vi "SGSA_Power_Freq_Sweep_Only_ELTA.vi"() -> ()   [LabVIEW 2023, in "SG_SA.lvlib"]
uses:
  SG_SA.lvlib
  lib/Keysight/Keysight.lvlib
panel:
  out "SA Freq(MHz)":i32
  out "SG Freq(MHz)":i32
  out "[SA]_Loss":dbl=8.0
  out "[SG]_Loss":dbl=8.0
  out "SG Power":i32
  in  "[SA] -> DUT Loss\nFreq.(MHz)          Loss":dbl[][](array[numeric])
  in  "[SG] -> DUT Loss\nFreq.(MHz)       Loss":dbl[][](array[numeric])
  in  "Waiting Time(ms)":u32=100
  in  "Stop Power":i32=18
  in  "Start Power":i32=-20
  in  "AvgTimes":i32=5
  in  "FileNote":string
  in  "SG":refnum<visa-resource-name>="TCPIP0::192.168.100.201::inst0::INSTR"
  in  "SA":refnum<visa-resource-name>="TCPIP0::192.168.100.202::inst0::INSTR"
  out "Spectrum Data":cluster{"X":dbl, "Y":dbl}[](graph)
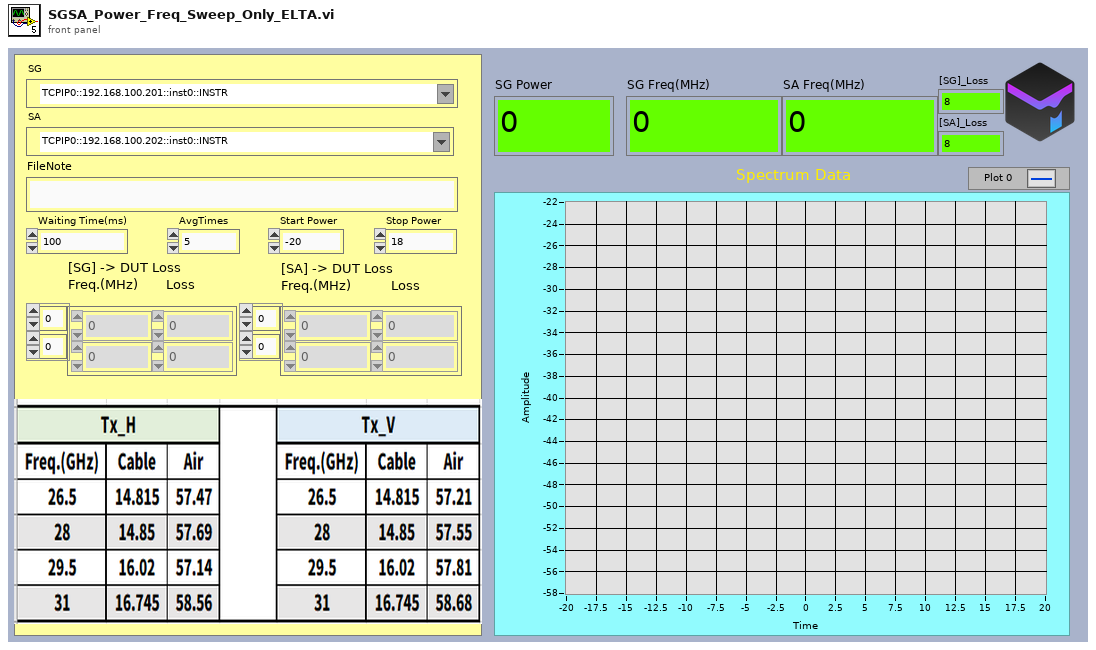
[diagram p1: front panel]
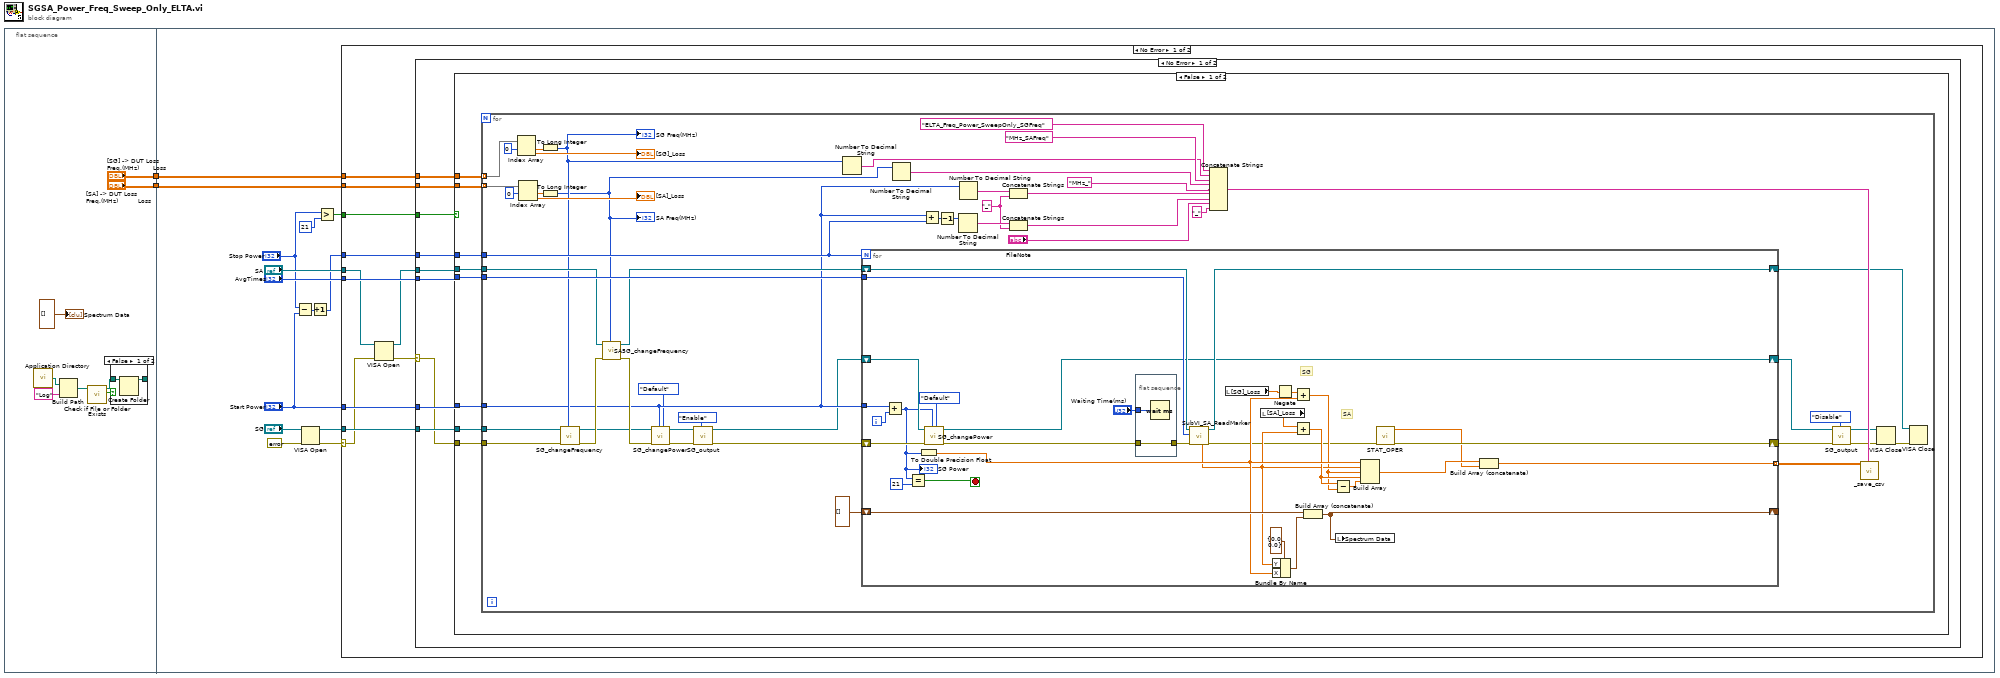
[diagram p0: block diagram]
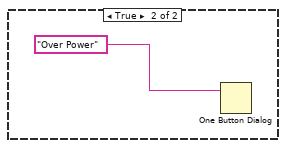
[diagram p3: hidden frame]
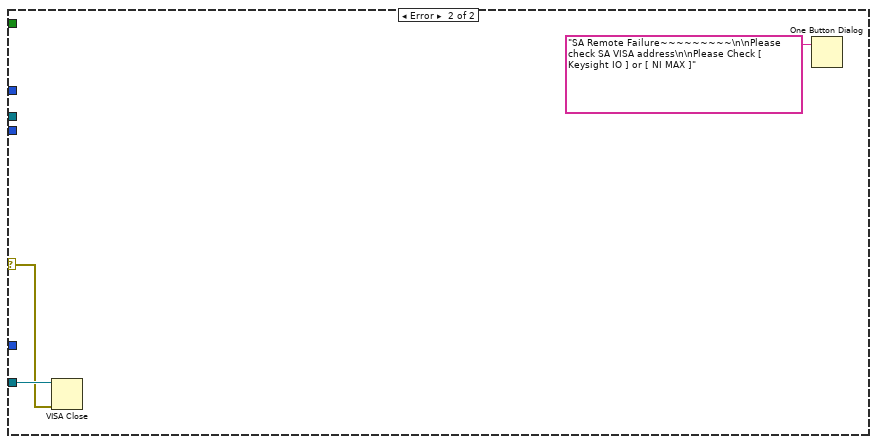
[diagram p4: hidden frame]
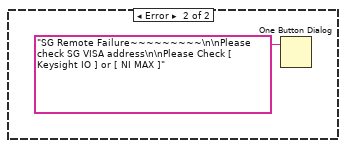
[diagram p5: hidden frame]
diagram:
  n1 = flat-sequence {
    tunnel: ["[SA] -> DUT Loss\nFreq.(MHz)          Loss"] -> w2
    tunnel: ["[SG] -> DUT Loss\nFreq.(MHz)       Loss"] -> w1
    tunnel: w2 -> [w15]
    tunnel: w1 -> [w14]
    frame #0 {
      n2 = call <vilib>:"Application Directory.vi"() -> ("Application Directory"=w9:path)
      n3 = Build Path(base path=w9, name or relative path="Log") -> (appended path=w6:path)
      n4 = call <vilib>:"Check if File or Folder Exists.vi"("path"=w6) -> ("file or folder exists?"=w8:bool, "dup path"=w7:path)  [unwired: 8 in, 1 out]
      n5 = case shown="False" w8 {
        tunnel: w7 -> [w12 w13]
        tunnel: [w11 w13] -> _
        frame False {
          n6 = Create Folder(path (use dialog)=w12) -> (created path=w11:path)  [unwired: 2 in, 2 out]
        }
        frame True {
        }
      }
      "Spectrum Data" <- cluster{"X":dbl, "Y":dbl}[] [] ("XY Graph")
    }
    frame #1 {
      n7 = Subtract(x="Stop Power", y="Start Power") -> (x-y=w23:i32)
      n8 = VISA Open(error in (no error)=errorcluster {"status"=FALSE, "code"=0, "source"=""}, VISA resource name="SG") -> (VISA resource name=w17:refnum<visa-resource-name>, error out=w16:errorcluster)  [unwired: 3 in]
      n9 = Increment(x=w23) -> (x+1=w22:i32)
      n10 = Greater?(x="Stop Power", y=21) -> (0:w26:bool)
      n11 = case shown="No Error" w16 {
        selector: w16 -> [w33 _]
        tunnel: "SA" -> [w31 _]
        tunnel: w26 -> [w38 _]
        tunnel: "Start Power" -> [w37 _]
        tunnel: "AvgTimes" -> [w36 _]
        tunnel: w22 -> [w35 _]
        tunnel: w17 -> [w34 _]
        tunnel: w15 -> [w29 _]
        tunnel: w14 -> [w28 _]
        frame No Error {
          n12 = VISA Open(error in (no error)=w33, VISA resource name=w31) -> (VISA resource name=w30:refnum<visa-resource-name>, error out=w32:errorcluster)  [unwired: 3 in]
          n13 = case shown="No Error" w32 {
            selector: w32 -> [w41 w141]
            tunnel: w30 -> [w47 _]
            tunnel: w38 -> [w46 _]
            tunnel: w37 -> [w45 _]
            tunnel: w36 -> [w44 _]
            tunnel: w35 -> [w43 _]
            tunnel: w34 -> [w42 w142]
            tunnel: w29 -> [w40 _]
            tunnel: w28 -> [w39 _]
            frame No Error {
              n14 = case shown="False" w46 {
                tunnel: w47 -> [w55 _]
                tunnel: w44 -> [w54 _]
                tunnel: w45 -> [w51 _]
                tunnel: w41 -> [w53 _]
                tunnel: w42 -> [w52 _]
                tunnel: w43 -> [w50 _]
                tunnel: w40 -> [w49 _]
                tunnel: w39 -> [w48 _]
                frame False {
                  n15 = for {
                    tunnel: w55 -> [w77]
                    tunnel: w54 -> [w105]
                    tunnel: w53 -> [w82]
                    tunnel: w52 -> [w81]
                    tunnel: w51 -> [w67]
                    tunnel: w50 -> [w96]
                    tunnel: w49 -> [w86] mode=indexing
                    tunnel: w48 -> [w89] mode=indexing
                    w100 = "_"
                    n16 = Index Array(array=w89, index #1=0 ("index")) -> (element #1=w80:dbl, element #2=→"[SG]_Loss":dbl)  [unwired: 1 in]
                    n17 = Index Array(array=w86, index #1=0 ("index")) -> (element #1=w79:dbl, element #2=→"[SA]_Loss":dbl)  [unwired: 1 in]
                    n18 = To Long Integer(number=w80) -> (32bit integer=w71:i32)
                    "SG Freq(MHz)" <- w71
                    n19 = To Long Integer(number=w79) -> (32bit integer=w70:i32)
                    "SA Freq(MHz)" <- w70
                    n20 = call "SG_changeFrequency.vi"("MHz"=w71, "error in"=w82, "VISA in"=w81) -> ("error out"=w83:errorcluster, "VISA out"=w68:refnum<visa-resource-name>)  [unwired: 6 in, 1 out]
                    n21 = call "SA5G_changeFrequency.vi"("MHz"=w70, "error in"=w83, "VISA in"=w77) -> ("error out"=w69:errorcluster, "VISA out"=w78:refnum<visa-resource-name>)  [unwired: 6 in, 1 out]
                    n22 = call "SG_changePower.vi"("Type"=enum16{"Default", "E6680A"}."Default", "dBm"=w67, "error in"=w69, "VISA in"=w68) -> ("error out"=w64:errorcluster, "VISA out"=w65:refnum<visa-resource-name>)  [unwired: 5 in, 1 out]
                    n23 = call "SG_output.vi"("Func."=enum16{"Disable", "Enable"}."Enable", "error in"=w64, "VISA in"=w65) -> ("error out"=w61:errorcluster, "VISA out"=w62:refnum<visa-resource-name>)  [unwired: 7 in]
                    n24 = Number To Decimal String(number=w71) -> (decimal integer string=w73:string)  [unwired: 1 in]
                    n25 = for {
                      N: w96 -> [_]
                      tunnel: w105 -> [w136]
                      tunnel: w67 -> [w134]
                      shift-right: [w109] -> w60
                      shift-left: w61 -> [w116]
                      shift-right: [w114] -> w59
                      shift-left: w62 -> [w113]
                      tunnel: [w107] -> w93 mode=indexing
                      shift-right: [w129] -> w90
                      shift-left: w78 -> [w137]
                      shift-right: [w125] -> _
                      shift-left: cluster{"X":dbl, "Y":dbl}[] [] ("XY Graph") -> [w127]
                      i -> [w135]
                      stop <- w132 stop-if-true
                      # "SA"
                      # "SG"
                      n26 = Add(x=w134, y=w135) -> (x+y=w112:i32)
                      "SG Power" <- w112
                      n27 = Equal?(x=w112, y=21) -> (x = y?=w132:bool)
                      n28 = To Double Precision Float(number=w112) -> (double precision float=w124:dbl)
                      n29 = call "SG_changePower.vi"("Type"=enum16{"Default", "E6680A"}."Default", "dBm"=w112, "error in"=w116, "VISA in"=w113) -> ("error out"=w115:errorcluster, "VISA out"=w114:refnum<visa-resource-name>)  [unwired: 5 in, 1 out]
                      n30 = flat-sequence {
                        tunnel: w115 -> [w139]
                        tunnel: [w139] -> w131
                        tunnel: "Waiting Time(ms)" -> [w138]
                        frame #0 {
                          n31 = Wait (ms)(milliseconds to wait=w138) -> ()  [unwired: 1 out]
                        }
                      }
                      n32 = call "SubVI_SA_ReadMarker.vi"("error in (no error)"=w131, "AvgTimes"=w136, "VISA resource name"=w137) -> ("error out"=w110:errorcluster, "VISA resource name out"=w129:refnum<visa-resource-name>, "Marker Power"=w122:dbl)  [unwired: 5 in, 1 out]
                      n33 = local read "[SG]_Loss"() -> (w118:dbl)
                      n34 = local read "[SA]_Loss"() -> (w117:dbl)
                      n35 = Bundle By Name(cluster=cluster{"X":dbl, "Y":dbl} {"X"=0.0, "Y"=0.0} ("element"), "Y"=w122, "X"=w124) -> (w126:cluster{"X":dbl, "Y":dbl})
                      n36 = Negate(x=w118) -> (-x=w119:dbl)
                      n37 = Add(x=w119, y=w124) -> (x+y=w121:dbl)
                      n38 = Add(x=w117, y=w122) -> (x+y=w123:dbl)
                      n39 = Build Array (concatenate)(w127, w126) -> (w125:cluster{"X":dbl, "Y":dbl}[])
                      n40 = Subtract(x=w123, y=w121) -> (x-y=w120:dbl)
                      n41 = local write "Spectrum Data"(w125) -> ()
                      n42 = Build Array(w124, w122, w121, w123, w120) -> (w108:dbl[])
                      n43 = call "STAT_OPER.vi"("error in"=w110) -> ("error out"=w109:errorcluster, "f_all_data"=w106:dbl[])  [unwired: 9 in]
                      n44 = Build Array (concatenate)(w108, w106) -> (w107:dbl[])
                    }
                    n45 = Number To Decimal String(number=w70) -> (decimal integer string=w75:string)  [unwired: 1 in]
                    n46 = Add(x=w67, y=w96) -> (x+y=w104:i32)
                    n47 = Decrement(x=w104) -> (x-1=w103:i32)
                    n48 = Number To Decimal String(number=w103) -> (decimal integer string=w101:string)  [unwired: 1 in]
                    n49 = Number To Decimal String(number=w67) -> (decimal integer string=w102:string)  [unwired: 1 in]
                    n50 = Concatenate Strings(w102, w100) -> (w99:string)
                    n51 = Concatenate Strings(w101, w100) -> (w98:string)
                    n52 = Concatenate Strings("ELTA_Freq_Power_SweepOnly_SGFreq" ("delimiter (\\t)"), w73, "MHz_SAFreq", w75, "MHz_", w99, w98, "FileNote", "_") -> (w97:string)
                    n53 = call "SG_output.vi"("Func."=enum16{"Disable", "Enable"}."Disable", "error in"=w60, "VISA in"=w59) -> ("error out"=w57:errorcluster, "VISA out"=w58:refnum<visa-resource-name>)  [unwired: 7 in]
                    n54 = call "_save_csv.vi"("delimiter (\\t)"=w97, "Data"=w93) -> ()  [unwired: 9 in, 1 out]
                    n55 = VISA Close(VISA resource name=w58, error in (no error)=w57) -> (error out=w91:errorcluster)
                    n56 = VISA Close(VISA resource name=w90, error in (no error)=w91) -> ()  [unwired: 1 out]
                  }
                }
                frame True {
                  n57 = One Button Dialog(message="Over Power") -> ()  [unwired: 1 in, 1 out]
                }
              }
            }
            frame Error {
              n58 = VISA Close(VISA resource name=w142, error in (no error)=w141) -> ()  [unwired: 1 out]
              n59 = One Button Dialog(message="SA Remote Failure~~~~~~~~~\n\nPlease check SA VISA address\n\nPlease Check [ Keysight IO ] or [ NI MAX ]") -> ()  [unwired: 1 in, 1 out]
            }
          }
        }
        frame Error {
          n60 = One Button Dialog(message="SG Remote Failure~~~~~~~~~\n\nPlease check SG VISA address\n\nPlease Check [ Keysight IO ] or [ NI MAX ]") -> ()  [unwired: 1 in, 1 out]
        }
      }
    }
  }
